vi "create new channel.vi"(8 "error in (no error)":errorcluster, 9 "channel info":T1, 10 "id":string, 11 "DSFConfiguration in":refnum<class "DSFConfiguration.lvclass">) -> (0 "error out":errorcluster, 3 "DSFConfiguration out":refnum<class "DSFConfiguration.lvclass">)   [LabVIEW 2017, in "DSFConfiguration.lvclass"]
uses:
  DSFConfiguration.lvclass
  Controls/dsf channel.ctl
  DSFConfiguration.lvclass/DSFConfiguration.ctl
  DSFChannel/DSFChannel.lvclass
  C:/github/data-sharing-framework/Source/Configuration API/Classes/IDable/IDable.lvclass
  IDable/IDable.lvclass/IDable.ctl
  IDable/Write id.vi
  <vilib>/Utility/error.llb/Error Cluster From Error Code.vi
  <vilib>/ErrorRing/Error Ring.xnode
  ID API/ID API.lvclass
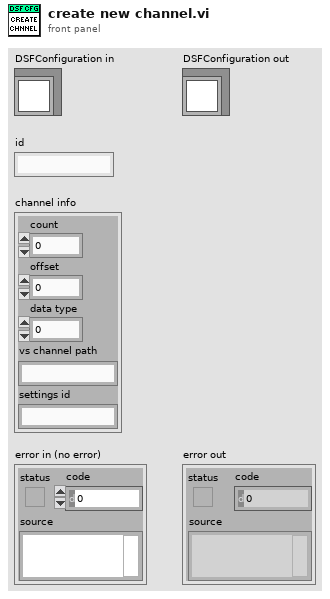
[diagram p1: front panel]
types:
  T1 = typedef "dsf channel.ctl" = cluster{"count":i32, "offset":i32, "data type":i32, "vs channel path":string, "settings id":string}
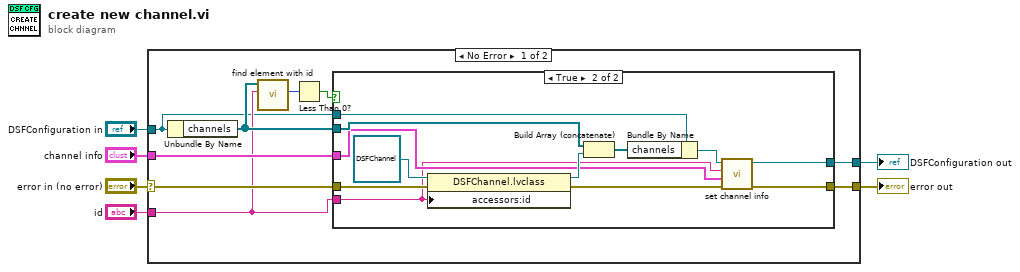
[diagram p0: block diagram]
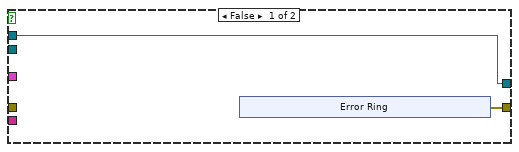
[diagram p2: hidden frame]
diagram:
  n1 = case shown="No Error" "error in (no error)" {
    selector: "error in (no error)" -> [w11 w35]
    tunnel: [w12 w35] -> w5
    tunnel: "DSFConfiguration in" -> [w7 w34]
    tunnel: "id" -> [w9 _]
    tunnel: "channel info" -> [w10 _]
    tunnel: [w8 w34] -> w1
    frame No Error {
      n2 = Unbundle By Name(w7) -> ("channels"=w13:refnum<class "DSFChannel.lvclass">[])
      n3 = call "find element with id.vi"("id"=w9, "IDable Array in"=w13) -> ("index"=w15:i32)  [unwired: 8 in, 1 out]
      n4 = Less Than 0?(x=w15) -> (x < 0?=w14:bool)
      n5 = case shown="True" w14 {
        tunnel: w13 -> [_ w33]
        tunnel: [w17 w24] -> w12
        tunnel: w11 -> [_ w32]
        tunnel: w10 -> [_ w23]
        tunnel: w9 -> [_ w22]
        tunnel: w7 -> [w16 w29]
        tunnel: [w16 w25] -> w8
        frame False {
          n6 = xnode "Error Ring"() -> ("error out"=w17:errorcluster)
        }
        frame True {
          n7 = property class="DSFChannel.lvclass"(reference=refnum<class "DSFChannel.lvclass"> refnum ("DSFChannel.lvclass"), error in=w32, "accessors:id"=w22) -> (reference out=w30:refnum<class "DSFChannel.lvclass">, error out=w26:errorcluster)
          n8 = Build Array (concatenate)(w33, w30) -> (w28:refnum<class "DSFChannel.lvclass">[])
          n9 = Bundle By Name(cluster=w29, "channels"=w28) -> (w27:refnum<class "DSFConfiguration.lvclass">)
          n10 = call "set channel info.vi"("error in (no error)"=w26, "channel info"=w23, "id"=w22, "DSFConfiguration in"=w27) -> ("error out"=w24:errorcluster, "DSFConfiguration out"=w25:refnum<class "DSFConfiguration.lvclass">)  [unwired: 6 in]
        }
      }
    }
    frame Error {
    }
  }
  "error out" <- w5
  "DSFConfiguration out" <- w1
